vi "Create Groups.vi"(7 "Group":bool, 8 "error in (no error)":errorcluster, 11 "Channels":T1[](array[typedef]) {"Data Type" format="%.0x"}) -> (0 "error out":errorcluster, 3 "Channels out":T1[](array[typedef]) {"Data Type" format="%.0x"})   [LabVIEW 2019, in "FPGA Addon System Explorer.lvlib"]
uses:
  FPGA Addon System Explorer.lvlib
  Addon Shared/Types/Register Information.ctl
  Addon Shared/Types/Data Type.ctl
  Addon Shared/FPGA Addon Shared.lvlib
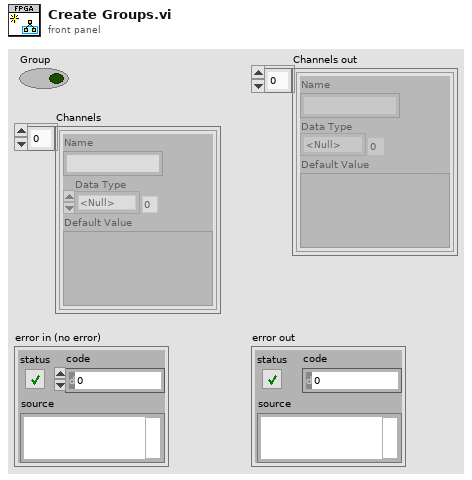
[diagram p1: front panel]
types:
  T1 = typedef "FPGA Addon Shared.lvlib/Register Information.ctl" = cluster{"Name":string, "Data Type":T2, "Default Value":variant}
  T2 = typedef "FPGA Addon Shared.lvlib/Data Type.ctl" = enum8{"<Null>", "I8", "I16", "I32", "I64", "U8", "U16", "U32", "U64", "SGL", "Boolean", "Analog PWM In Settings", "Analog PWM In", "Digital PWM In Settings", "Digital PWM In", "Digital PWM Out", "Sine Out", "FXP+/-24.5", "FXP+/-16.5", "FXP+/-32.8", "FXP+/-64.32", "FXP+/-16.7", "FXP+/-20.5", "FXP+/-27.5", "FXP+/-32.16", "FXP+16.3", "FXP+18.3", "Digital Static In", "Digital Static Out", "Digital Static In Settings", "Digital WSS Out", "Quad Encoder Settings", "Quad Encoder In", "Group"}
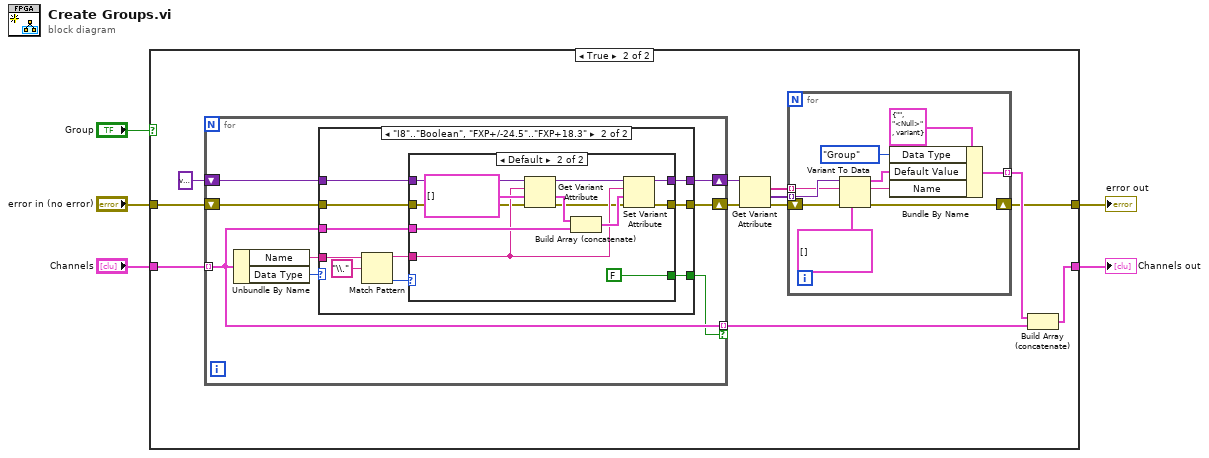
[diagram p0: block diagram]
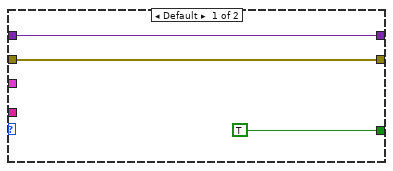
[diagram p3: hidden frame]
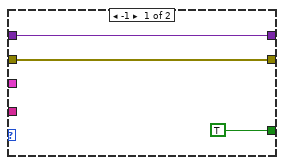
[diagram p4: hidden frame]
diagram:
  n1 = case shown="True" "Group" {
    tunnel: "Channels" -> [w6 w19]
    tunnel: "error in (no error)" -> [w7 w10]
    tunnel: [w7 w9] -> w3
    tunnel: [w6 w8] -> w5
    frame False {
    }
    frame True {
      n2 = for {
        tunnel: w19 -> [w32] mode=indexing
        shift-right: [w33] -> w17
        shift-left: variant -> [w34]
        tunnel: [w32] -> w11 mode=indexing if=w31
        shift-right: [w30] -> w14
        shift-left: w10 -> [w29]
        n3 = Unbundle By Name(w32) -> ("Name"=w36:string, "Data Type"=w35:T2)
        n4 = case shown="\"I8\"..\"Boolean\", \"FXP+/-24.5\"..\"FXP+18.3\"" w35 {
          tunnel: w36 -> [_ w49]
          tunnel: w34 -> [w39 w46]
          tunnel: w32 -> [_ w44]
          tunnel: [w39 w43] -> w33
          tunnel: [TRUE w42] -> w31
          tunnel: [w37 w41] -> w30
          tunnel: w29 -> [w37 w40]
          frame Default {
          }
          frame "I8".."Boolean", "FXP+/-24.5".."FXP+18.3" {
            n5 = Match Pattern(string=w49, regular expression="\\.") -> (before substring=w45:string, offset past match=w47:i32)  [unwired: 1 in, 2 out]
            n6 = case shown="Default" w47 {
              tunnel: w46 -> [w52 w64]
              tunnel: w45 -> [_ w59]
              tunnel: w44 -> [_ w61]
              tunnel: [w52 w58] -> w43
              tunnel: [TRUE FALSE] -> w42
              tunnel: [w50 w56] -> w41
              tunnel: w40 -> [w50 w55]
              frame -1 {
              }
              frame Default {
                n7 = Get Variant Attribute(Variant=w64, name=w59, default value (empty Variant)=T1[] [], error in=w55) -> (duplicate Variant=w53:variant, value=w62:T1[], error out=w54:errorcluster)  [unwired: 1 out]
                n8 = Build Array (concatenate)(w62, w61) -> (w60:T1[])
                n9 = Set Variant Attribute(Variant=w53, name=w59, value=w60, error in=w54) -> (Variant out=w58:variant, error out=w56:errorcluster)  [unwired: 1 out]
              }
            }
          }
        }
      }
      n10 = Get Variant Attribute(Variant=w17, error in=w14) -> (names=w16:string[], values=w15:variant[], error out=w13:errorcluster)  [unwired: 2 in, 1 out]
      n11 = for {
        tunnel: w16 -> [w20] mode=indexing
        tunnel: w15 -> [w28] mode=indexing
        tunnel: [w23] -> w12 mode=indexing
        shift-right: [w21] -> w9
        shift-left: w13 -> [w22]
        n12 = Variant To Data(error in=w22, type=T1[] [], Variant=w28) -> (data=w24:T1[], error out=w21:errorcluster)
        n13 = Bundle By Name(cluster=T1 {"Name"="", "Data Type"=enum."<Null>", "Default Value"=variant}, "Data Type"=Data_Type."Group", "Default Value"=w24, "Name"=w20) -> (w23:T1)
      }
      n14 = Build Array (concatenate)(w12, w11) -> (w8:T1[])
    }
  }
  "Channels out" <- w5
  "error out" <- w3
